vi "Revert User Dialog.vi"(8 "error in (no error)":errorcluster) -> (0 "error out":errorcluster, 2 "Revert":bool)   [LabVIEW 2021, in "Script gRPC.lvlib"]
uses:
  Script gRPC.lvlib
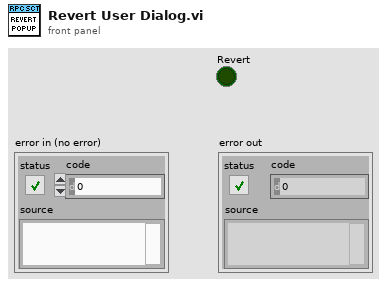
[diagram p1: front panel]
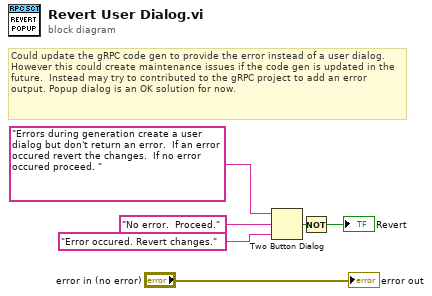
[diagram p0: block diagram]
diagram:
  # "Could update the gRPC code gen to provide the error instead of a user dialog.  However this could create maintenance issues if the code gen is updated in the future.  Instead may try to contributed to the gRPC project to add an error output. Popup dialog is an OK solution for now."
  n1 = Two Button Dialog(message="Errors during generation create a user dialog but don't return an error.  If an error occured revert the changes.  If no error occured proceed. ", 1:"Error occured. Revert changes." ("F button name (\"Cancel\")"), 2:"No error.  Proceed." ("T button name (\"OK\")")) -> (T button?=w3:bool)
  n2 = Not(x=w3) -> (.not. x?=→"Revert":bool)
  "error out" <- "error in (no error)"
